vi "Set_Traverse_Position.vi"(3 "Simulate/Run":T3, 4 "Currently on Point":i32=11, 5 "Traverse line":T4 {"Row Duration (mins)" format="%#.1f"; "Row No" min=0; "Trace Gas Concentration (%)" min=0.0 format="%#.2f"; "Emission Rate (l/min)" format="%#.2f"; "Tunnel Speed" format="%#.2f"; "Start X" format="%#.2f"; "Start Y" format="%#.2f"; "Start Z" format="%#.2f"; "End X" format="%#.2f"; "End Y" format="%#.2f"; "End Z" format="%#.2f"; "Averaging time (min)" min=0.0 format="%#.2f"}) -> (0 "Status Cluster":T1)   [LabVIEW 2013]
uses:
  Traverse_cluster.ctl
  Spacing.ctl
  Controls/Multi_run_mode.ctl
  Controls/User_Specific_mode.ctl
  Status_Cluster.ctl
  Multi_Run_Status.ctl
  Trav_mode.ctl
  Globals/Dynamic_call_global.ph.vi
  Globals/Constants_global.vi
panel:
  # "X           Y            Z"
  # "Start"
  # "End"
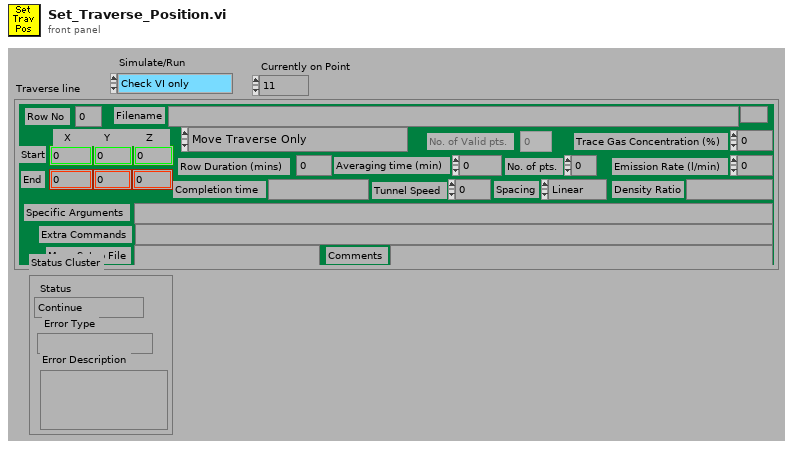
[diagram p1: front panel]
types:
  T1 = typedef "Status_Cluster.ctl" = cluster{"Status":T2, "Error Type":string, "Error Description":string}
  T2 = typedef "Multi_Run_Status.ctl" = enum16{"Continue", "Jump to Next Point", "Jump to Next Row", "Jump To Fall Back", "Terminate Run"}
  T3 = typedef "User_Specific_mode.ctl" = enum16{"Check VI only", "Run VI"}
  T4 = typedef "Traverse_cluster.ctl" = cluster{"Start X":dbl, "Start Y":dbl, "Start Z":dbl, "End X":dbl, "End Y":dbl, "End Z":dbl, "No. of pts.":i32, "Spacing":T5, "Filename":path, "Tunnel Speed":dbl, "Averaging time (min)":dbl, "Extra Commands":string, "Specific Arguments":string, "Emission Rate (l/min)":dbl, "Trace Gas Concentration (%)":dbl, "Density Ratio":string, "Comments":string, "Row No":i32, "Row Type Selector":T6, "Completion time":string, "Row Duration (mins)":dbl, "No. of Valid pts.":i32, "Meas Setup File":string}
  T5 = typedef "Spacing.ctl" = enum16{"Linear", "Log", "Gauss", "Specified", "N/A"}
  T6 = typedef "Multi_run_mode.ctl" = enum16{"Move Traverse Only", "Set Tunnel Speed Only", "Set Source Only", "Set Measurement Conditions", "Single Measurement", "Vertical Profile", "Lateral Profile", "Longitudinal Profile", "Explore Volume", "Multi-Axis Profile", "Auto Calibrate", "Meas Fast FID Bkgnd", "Check Beam Power", "Scanning Valve Measurement", "Run VI Named:", "Set ADAM Ch", "Wait (minutes)", "Send Message", "Synchronize With:", "Fall Back to this Row", "Turn Off Row Repeating", "Blank Row", "Traverse 3D Volume"}
  T7 = typedef "Trav_mode.ctl" = enum16{"Move traverse", "Read traverse position", "Teach Position"}
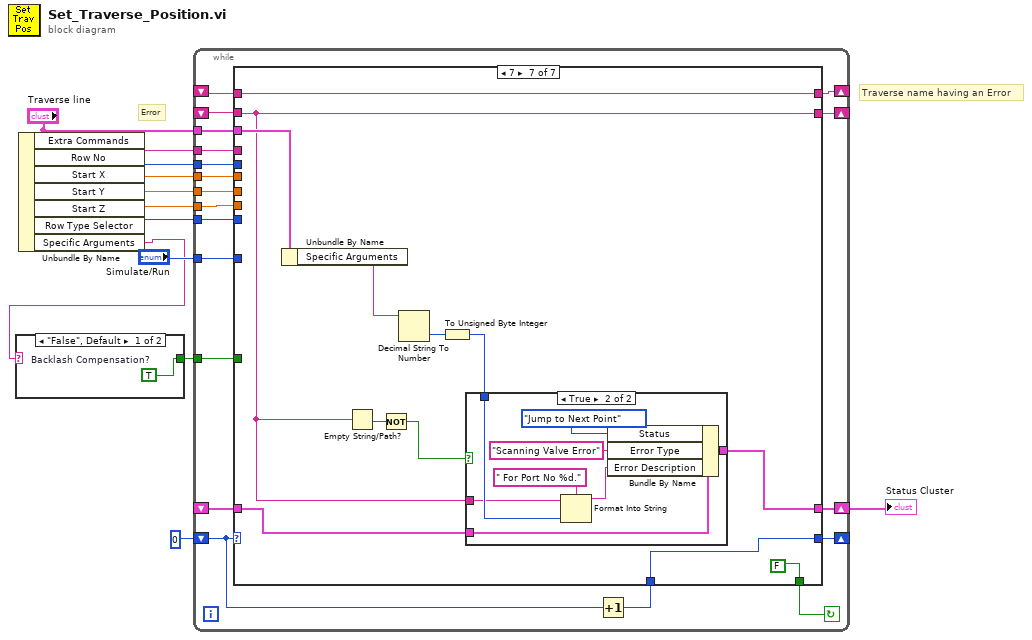
[diagram p0: block diagram]
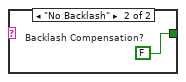
[diagram p2: hidden frame]
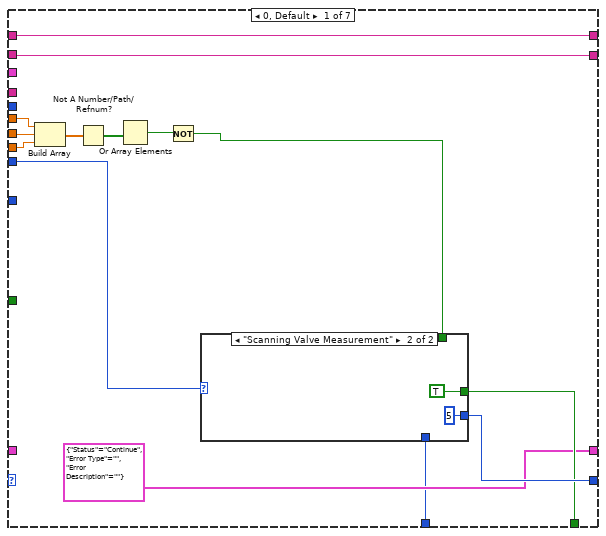
[diagram p3: hidden frame]
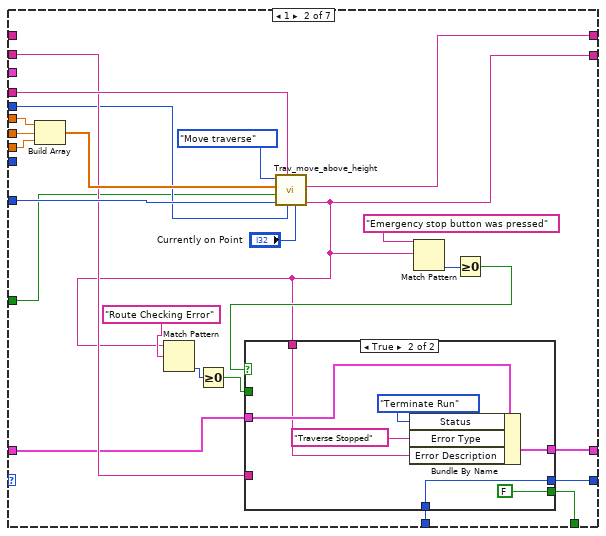
[diagram p5: hidden frame]
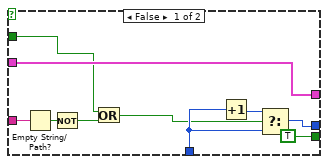
[diagram p6: hidden frame]
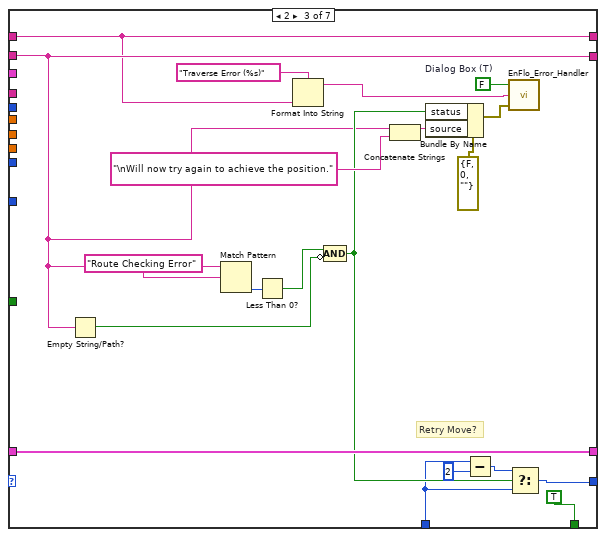
[diagram p7: hidden frame]
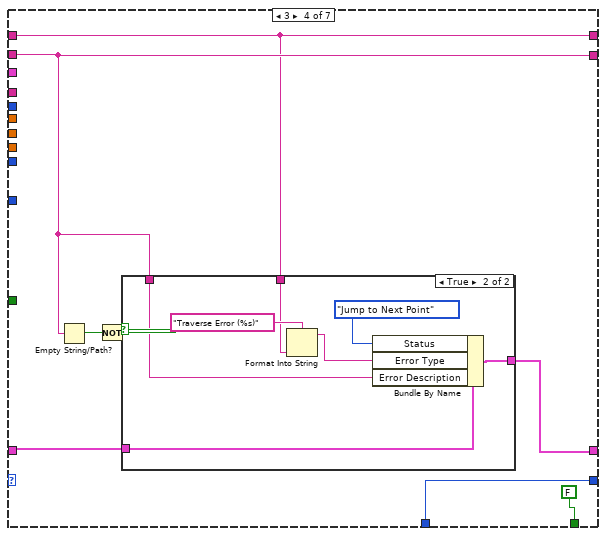
[diagram p8: hidden frame]
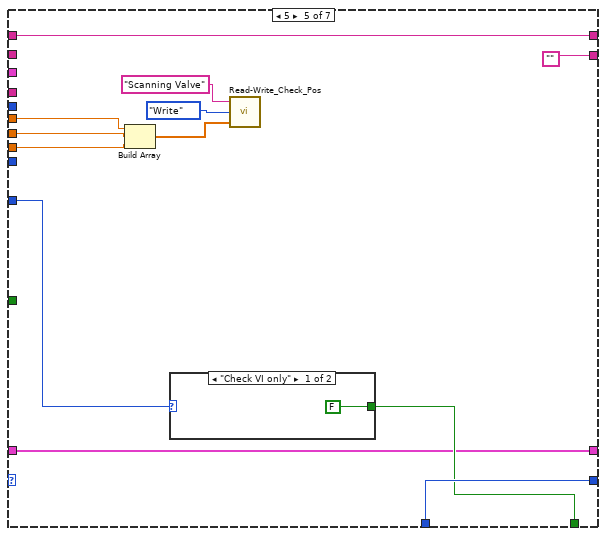
[diagram p10: hidden frame]
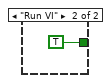
[diagram p11: hidden frame]
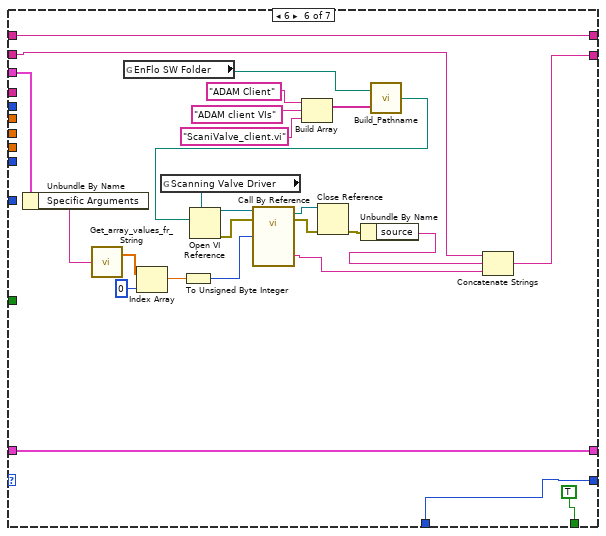
[diagram p12: hidden frame]
diagram:
  # "Traverse name having an Error"
  # "Error"
  n1 = Unbundle By Name("Traverse line") -> ("Extra Commands"=w11:string, "Row No"=w10:i32, "Start X"=w7:dbl, "Start Y"=w12:dbl, "Start Z"=w6:dbl, "Row Type Selector"=w8:T6, "Specific Arguments"=w2:string)
  n2 = case shown="\"False\", Default" w2 {
    tunnel: [w13 w14] -> w1
    frame "False", Default {
      w13 = TRUE  # Backlash Compensation?
    }
    frame "No Backlash" {
      w14 = FALSE  # Backlash Compensation?
    }
  }
  n3 = while {
    shift-left: _ -> [w18]
    shift-right: [w19] -> _
    shift-left: _ -> [w20]
    shift-right: [w21] -> w3
    tunnel: "Traverse line" -> [w22]
    tunnel: "Simulate/Run" -> [w23]
    tunnel: w6 -> [w24]
    tunnel: w12 -> [w25]
    tunnel: w7 -> [w26]
    tunnel: w8 -> [w31]
    shift-left: 0 -> [w29]
    shift-right: [w28] -> _
    tunnel: w10 -> [w32]
    tunnel: w11 -> [w33]
    tunnel: w1 -> [w17]
    shift-right: [w16] -> _
    shift-left: _ -> [w15]
    stop <- w30 continue-if-true
    n4 = Increment(x=w29) -> (x+1=w27:i32)
    n5 = case shown="7" w29 {
      tunnel: w33 -> [_ w73 _ _ _ _ _]
      tunnel: w32 -> [_ w64 _ _ _ _ _]
      tunnel: w31 -> [w47 _ _ _ _ _ _]
      tunnel: [w45 w58 TRUE FALSE w138 TRUE FALSE] -> w30
      tunnel: [w46 w66 w98 w118 w140 w145 w170] -> w28
      tunnel: w27 -> [w43 w67 w99 w118 w140 w145 w170]
      tunnel: w26 -> [w39 w72 _ _ w132 _ _]
      tunnel: w25 -> [w40 w71 _ _ w131 _ _]
      tunnel: w24 -> [w41 w70 _ _ w130 _ _]
      tunnel: w23 -> [_ w68 _ _ w139 _ _]
      tunnel: w22 -> [_ _ _ _ _ w162 w179]
      tunnel: [T1 {"Status"=enum."Continue", "Error Type"="", "Error Description"=""} ("Status Cluster") w60 w107 w119 w137 w153 w176] -> w21
      tunnel: w20 -> [_ w59 w107 w120 w137 w153 w177]
      tunnel: [w42 w56 w97 w115 "" w146 w171] -> w19
      tunnel: w18 -> [w42 w65 w97 w115 _ w144 w171]
      tunnel: w17 -> [_ w53 _ _ _ _ _]
      tunnel: [w34 w52 w93 w113 w129 w143 w169] -> w16
      tunnel: w15 -> [w34 _ w93 w113 w129 w143 w169]
      frame 0, Default {
        n6 = Build Array(w39, w40, w41) -> (w38:dbl[])
        n7 = Not A Number/Path/Refnum?(number/path/refnum=w38) -> (NaN/Path/Refnum?=w37:bool[])
        n8 = Or Array Elements(Boolean array=w37) -> (logical OR=w36:bool)
        n9 = Not(x=w36) -> (.not. x?=w35:bool)
        n10 = case shown="\"Scanning Valve Measurement\"" w47 {
          tunnel: [w48 5] -> w46
          tunnel: [w49 TRUE] -> w45
          tunnel: w35 -> [w49 _]
          tunnel: w43 -> [w48 _]
          frame "Move Traverse Only", Default {
          }
          frame "Scanning Valve Measurement" {
          }
        }
      }
      frame 1 {
        n11 = Build Array(w72, w71, w70) -> (w69:dbl[])
        n12 = call "Trav_move_above_height.vi"("Currently on Point"="Currently on Point", "Row Number"=w64, "Extra Command String"=w73, "Simulate/Run"=w68, "Backlash Compensation?"=w53, "New Position"=w69, "Mode"=Trav_mode."Move traverse") -> ("Error String"=w56:string, "Error from Traverse named"=w52:string)  [unwired: 1 in, 2 out]
        n13 = Match Pattern(string=w56, regular expression="Route Checking Error") -> (offset past match=w55:i32)  [unwired: 4 out]
        n14 = Greater Or Equal To 0?(x=w55) -> (x >= 0?=w54:bool)
        n15 = Match Pattern(string=w56, regular expression="Emergency stop button was pressed") -> (offset past match=w62:i32)  [unwired: 4 out]
        n16 = Greater Or Equal To 0?(x=w62) -> (x >= 0?=w61:bool)
        n17 = case shown="True" w61 {
          tunnel: w67 -> [w84 w87]
          tunnel: [w83 w87] -> w66
          tunnel: w65 -> [w81 _]
          tunnel: [w80 w89] -> w60
          tunnel: w59 -> [w80 w90]
          tunnel: w56 -> [_ w88]
          tunnel: [TRUE FALSE] -> w58
          tunnel: w54 -> [w77 _]
          frame False {
            n18 = Empty String/Path?(string/path=w81) -> (empty?=w82:bool)
            n19 = Not(x=w82) -> (.not. x?=w78:bool)
            n20 = Or(x=w77, y=w78) -> (x .or. y?=w76:bool)
            n21 = Increment(x=w84) -> (x+1=w85:i32)
            n22 = Select(t=w85, s=w76, f=w84) -> (s? t:f=w83:i32)
          }
          frame True {
            n23 = Bundle By Name(cluster=w90, "Status"=Multi_Run_Status."Terminate Run", "Error Type"="Traverse Stopped" ("t"), "Error Description"=w88) -> (w89:T1)
          }
        }
      }
      frame 2 {
        w110 = FALSE  # Dialog Box (T)
        # "Retry Move?"
        n24 = Empty String/Path?(string/path=w97) -> (empty?=w96:bool)
        n25 = Match Pattern(string=w97, regular expression="Route Checking Error" ("String to match")) -> (offset past match=w104:i32)  [unwired: 4 out]
        n26 = Less Than 0?(x=w104) -> (x < 0?=w103:bool)
        n27 = Format Into String(format string="Traverse Error (%s)" ("t"), w93) -> (resulting string=w94:string)  [unwired: 2 in, 1 out]
        n28 = Compound Arithmetic op=AND(w103, invert w96) -> (w102:bool)
        n29 = Concatenate Strings(w97, "\nWill now try again to achieve the position." ("Substring")) -> (w109:string)
        n30 = Bundle By Name(cluster=errorcluster {"status"=FALSE, "code"=0, "source"=""} ("error in (no error)"), "status"=w102, "source"=w109) -> (w111:errorcluster)
        n31 = Subtract(x=w99, y=2) -> (x-y=w100:i32)
        n32 = call "EnFlo_Error_Handler.vi"("error in (no error)"=w111, "Error Type"=w94, "Dialog Box (T)"=w110) -> ()  [unwired: 3 out]
        n33 = Select(t=w100, s=w102, f=w99) -> (s? t:f=w98:i32)
      }
      frame 3 {
        n34 = Empty String/Path?(string/path=w115) -> (empty?=w116:bool)
        n35 = Not(x=w116) -> (.not. x?=w114:bool)
        n36 = case shown="True" w114 {
          tunnel: w120 -> [w121 w128]
          tunnel: [w121 w126] -> w119
          tunnel: w115 -> [_ w125]
          tunnel: w113 -> [_ w122]
          frame False {
          }
          frame True {
            n37 = Format Into String(format string="Traverse Error (%s)" ("t"), w122) -> (resulting string=w123:string)  [unwired: 2 in, 1 out]
            n38 = Bundle By Name(cluster=w128, "Status"=Multi_Run_Status."Jump to Next Point", "Error Type"=w123, "Error Description"=w125) -> (w126:T1)
          }
        }
      }
      frame 5 {
        n39 = Build Array(w132, w131, w130) -> (w135:dbl[])
        n40 = case shown="\"Check VI only\"" w139 {
          tunnel: [FALSE TRUE] -> w138
          frame "Check VI only" {
          }
          frame "Run VI" {
          }
        }
        n41 = call "Read-Write_Check_Pos.vi"("Position input"=w135, "Mode"=enum16{"Read", "Write"}."Write", "Traverse Name"="Scanning Valve") -> ()  [unwired: 1 out]
      }
      frame 6 {
        n42 = Unbundle By Name(w162) -> ("Specific Arguments"=w150:string)
        n43 = call "Get_array_values_fr_String.vi"("String Value"=w150) -> ("Numeric Array"=w152:dbl[])  [unwired: 1 out]
        n44 = global read "Constants_global.vi" "EnFlo SW Folder"() -> (w156:path)
        n45 = Index Array(array=w152, index=0) -> (element=w149:dbl)
        n46 = global read "Dynamic_call_global.ph.vi" "Scanning Valve Driver"() -> (w163:refnum<vi>)
        n47 = To Unsigned Byte Integer(number=w149) -> (unsigned 8bit integer=w161:u8)
        n48 = Build Array("ADAM Client", "ADAM client VIs", "ScaniValve_client.vi") -> (w157:string[])
        n49 = call "Build_Pathname.vi"("PathElements"=w157, "PathnameIn"=w156) -> ("AppendedPath"=w155:path)
        n50 = Open VI Reference(type specifier VI Refnum (for type only)=w163, vi path=w155) -> (vi reference=w164:refnum<vi>, error out=w165:errorcluster)  [unwired: 2 in, 2 out]
        n51 = call-by-ref "?"(reference=w164, error in=w165, "Port Number"=w161) -> (reference out=w167:refnum<vi>, error out=w166:errorcluster, "Error String"=w147:string)  [unwired: 2 out]
        n52 = Close Reference(reference=w167, error in (no error)=w166) -> (error out=w168:errorcluster)
        n53 = Unbundle By Name(w168) -> ("source"=w148:string)
        n54 = Concatenate Strings(w144, w148, w147) -> (w146:string)
      }
      frame 7 {
        n55 = Unbundle By Name(w179) -> ("Specific Arguments"=w180:string)
        n56 = Empty String/Path?(string/path=w171) -> (empty?=w173:bool)
        n57 = Not(x=w173) -> (.not. x?=w172:bool)
        n58 = Decimal String To Number(string=w180) -> (number=w178:i32)  [unwired: 3 out]
        n59 = To Unsigned Byte Integer(number=w178) -> (unsigned 8bit integer=w175:u8)
        n60 = case shown="True" w172 {
          tunnel: w177 -> [w181 w189]
          tunnel: [w181 w186] -> w176
          tunnel: w175 -> [_ w184]
          tunnel: w171 -> [_ w182]
          frame False {
          }
          frame True {
            n61 = Format Into String(format string=" For Port No %d." ("Format String"), initial string=w182, w184) -> (resulting string=w183:string)  [unwired: 1 in, 1 out]
            n62 = Bundle By Name(cluster=w189, "Status"=Multi_Run_Status."Jump to Next Point", "Error Type"="Scanning Valve Error" ("t"), "Error Description"=w183) -> (w186:T1)
          }
        }
      }
    }
  }
  "Status Cluster" <- w3
